vi "MemoryReport.vi"(10 "Channel Name":string, 11 "ProcessName":string) -> (2 "Comment":string, 3 "Reading":dbl format="%.3f")   [LabVIEW 2016]
panel:
  out "RSS":i32
  out "VSZ":i32
  out "CPU%":dbl
  out "Memory%":dbl
  out "CommandString":string
  out "standard error":string
  out "standard output":string
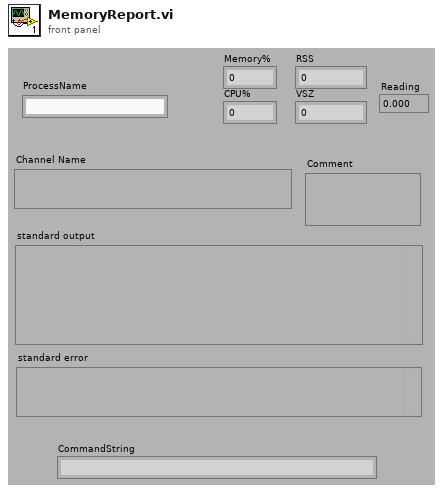
[diagram p1: front panel]
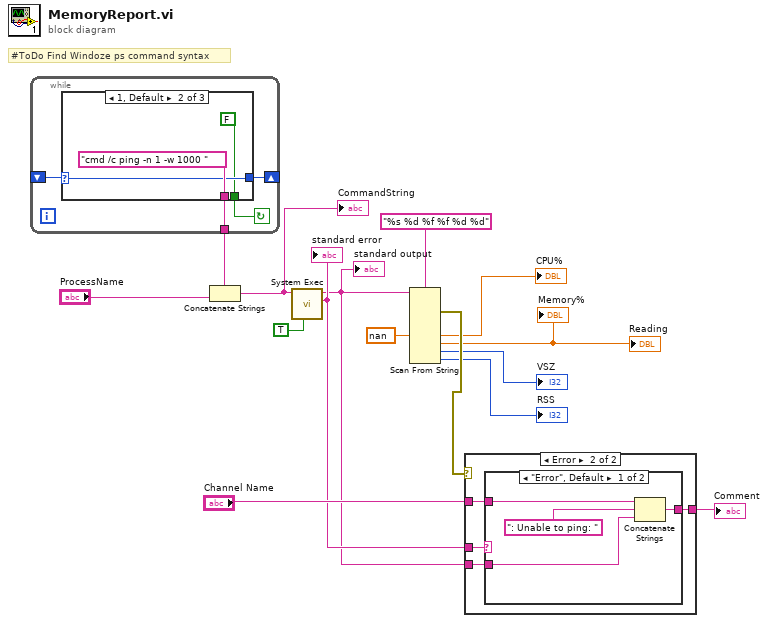
[diagram p0: block diagram]
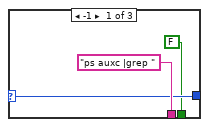
[diagram p2: hidden frame]
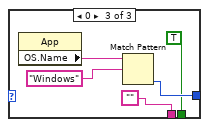
[diagram p3: hidden frame]
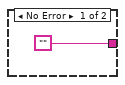
[diagram p4: hidden frame]
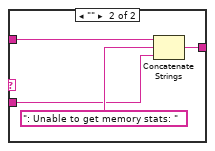
[diagram p5: hidden frame]
diagram:
  # "#ToDo Find Windoze ps command syntax"
  n1 = while {
    shift-right: [w18] -> _
    shift-left: _ -> [w19]
    tunnel: [w17] -> w11
    stop <- w16 continue-if-true
    n2 = case shown="1, Default" w19 {
      selector: w19 -> [w21 w24 _]
      tunnel: [w21 w24 w28] -> w18
      tunnel: ["ps auxc |grep " ("string") "cmd /c ping -n 1 -w 1000 " ("string") ""] -> w17
      tunnel: [FALSE FALSE TRUE] -> w16
      frame -1 {
      }
      frame 1, Default {
      }
      frame 0 {
        n3 = property class="App"() -> ("OS.Name"=w30:string)  [unwired: 2 in, 2 out]
        n4 = Match Pattern(string=w30, regular expression="Windows") -> (offset past match=w28:i32)  [unwired: 4 out]
      }
    }
  }
  n5 = Concatenate Strings(w11, "ProcessName") -> (w15:string)
  "CommandString" <- w15
  n6 = call <vilib>:"System Exec.vi"("run minimized? (F)"=TRUE, "command line"=w15) -> ("standard error"=w12:string, "standard output"=w8:string)  [unwired: 4 in, 4 out]
  "standard output" <- w8
  "standard error" <- w12
  n7 = Scan From String(format string="%s %d %f %f %d %d", input string=w8, default 3=nan ("default (0 dbl)")) -> (error out=w5:errorcluster, output 3=→"CPU%":dbl, output 4=→"Reading" →"Memory%":dbl, output 5=→"VSZ":i32, output 6=→"RSS":i32)  [unwired: 9 in, 2 out]
  n8 = case shown="Error" w5 {
    tunnel: w8 -> [_ w35]
    tunnel: ["" w34] -> w14
    tunnel: "Channel Name" -> [_ w33]
    tunnel: w12 -> [_ w32]
    frame No Error {
    }
    frame Error {
      n9 = case shown="\"Error\", Default" w32 {
        tunnel: w35 -> [w37 w42]
        tunnel: [w36 w41] -> w34
        tunnel: w33 -> [w38 w40]
        frame "Error", Default {
          n10 = Concatenate Strings(w38, ": Unable to ping: " ("string"), w37) -> (w36:string)
        }
        frame "" {
          n11 = Concatenate Strings(w40, ": Unable to get memory stats: " ("string"), w42) -> (w41:string)
        }
      }
    }
  }
  "Comment" <- w14
